vi "GetRegistry.vi"(8 "error in (no error)":errorcluster, 9 "data":T2, 11 "config":T1) -> (0 "error out":errorcluster, 1 "registry":T6)   [LabVIEW 2017, in "DataEventCreator.lvlib"]
uses:
  <vilib>/addons/InsightCM/Devices/Shared/Common/DataEventCreator/DataEventCreator.lvlib
  <vilib>/addons/InsightCM/Devices/Shared/Cms/CmsDataEventCreator/controls/GroupRegistry.ctl
  <vilib>/addons/InsightCM/Devices/Shared/Cms/CmsDataEventCreator/controls/DataSetRegistry.ctl
  <vilib>/addons/InsightCM/Devices/Shared/Common/DataEvent/controls/DataSetType.ctl
  <vilib>/addons/InsightCM/Devices/Shared/Common/DataEventCreator/controls/Registry_Trend.ctl
  <vilib>/addons/InsightCM/Devices/Shared/Common/DataFlow/controls/Data.ctl
  <vilib>/addons/InsightCM/Utilities/DataAccessors/controls/wfmSGL_DVR.ctl
  <vilib>/addons/PointValueMap/controls/PointMap.ctl
  <vilib>/addons/InsightCM/Devices/Shared/Common/DataFlow/controls/Type.ctl
  <vilib>/addons/InsightCM/Devices/Shared/Cms/CmsDataEventCreator/controls/config.ctl
  <vilib>/addons/InsightCM/Devices/Shared/Common/DataEvent/DataEvent.lvlib
  <vilib>/addons/InsightCM/Devices/Shared/Cms/CmsDataEventCreator/CmsDataEventCreator.lvlib
  <vilib>/addons/PointValueMap/PointValueMap.lvlib
  <vilib>/addons/InsightCM/Devices/Shared/Common/DataFlow/DataFlow.lvlib
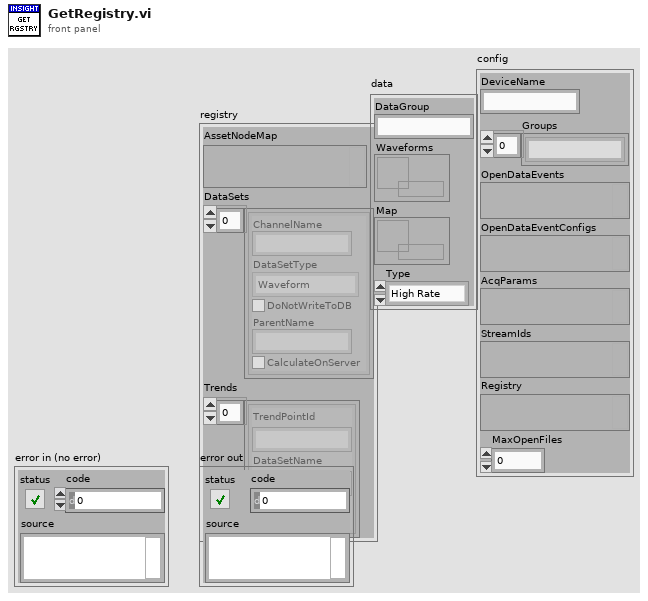
[diagram p1: front panel]
types:
  T1 = typedef "CmsDataEventCreator.lvlib/config.ctl" = cluster{"DeviceName":string, "Groups":string[], "OpenDataEvents":variant, "OpenDataEventConfigs":variant, "AcqParams":variant, "StreamIds":variant, "Registry":variant, "MaxOpenFiles":i32}
  T2 = typedef "DataFlow.lvlib/Data.ctl" = cluster{"DataGroup":string, "Waveforms":T3, "Map":T4, "Type":T5}
  T3 = typedef "wfmSGL_DVR.ctl" = refnum<data-value>
  T4 = typedef "PointValueMap.lvlib/PointMap.ctl" = refnum<data-value>
  T5 = typedef "DataFlow.lvlib/Type.ctl" = enum16{"High Rate", "Low Rate", "Burst Mode"}
  T6 = typedef "CmsDataEventCreator.lvlib/GroupRegistry.ctl" = cluster{"AssetNodeMap":variant, "DataSets":T7[], "Trends":T9[]}
  T7 = typedef "CmsDataEventCreator.lvlib/DataSetRegistry.ctl" = cluster{"ChannelName":string, "DataSetType":T8, "DoNotWriteToDB":bool, "ParentName":string, "CalculateOnServer":bool}
  T8 = typedef "DataEvent.lvlib/DataSetType.ctl" = enum16{"Waveform", "SpeedProfile", "ThermalImage", "EmsaSweep"}
  T9 = typedef "DataEventCreator.lvlib/Registry_Trend.ctl" = cluster{"TrendPointId":string, "DataSetName":string, "HighRate":bool, "Always Send":bool}
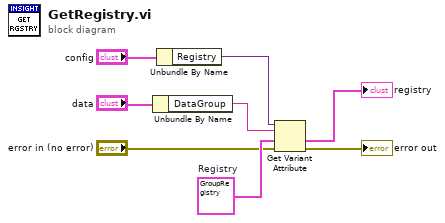
[diagram p0: block diagram]
diagram:
  w6 = T6 {"AssetNodeMap"=variant, "DataSets"=[], "Trends"=[]}  # Registry
  n1 = Unbundle By Name("data") -> ("DataGroup"=w3:string)
  n2 = Unbundle By Name("config") -> ("Registry"=w1:variant)
  n3 = Get Variant Attribute(Variant=w1, name=w3, default value (empty Variant)=w6, error in="error in (no error)") -> (value=→"registry":T6, error out=→"error out":errorcluster)  [unwired: 2 out]
